vi "SelectHandle.vi"(8 "error in (no error)":errorcluster, 11 "ClassIn":refnum<class "NISTFGenPluginsBase.lvclass">) -> (0 "error out":errorcluster, 3 "ClassOut":refnum<class "NISTFGenPluginsBase.lvclass">)   [LabVIEW 2014, in "FGenPlugins.lvlib" / "NISTFGenPluginsBase.lvclass"]
uses:
  NISTFGenPluginsBase.lvclass
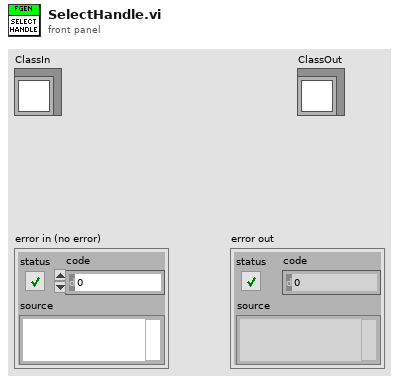
[diagram p1: front panel]
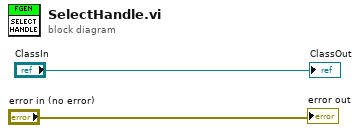
[diagram p0: block diagram]
diagram:
  "error out" <- "error in (no error)"
  "ClassOut" <- "ClassIn"
